vi "stage write_v2.vi"(3 "axis":u32, 4 "Incoming Handle":i32, 5 "position":dbl) -> (1 "out handle":i32)   [LabVIEW 2014]
uses:
  MCL-dll-Labview 32-bit/Madlib.dll
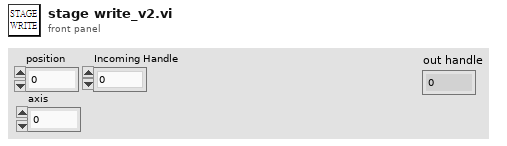
[diagram p1: front panel]
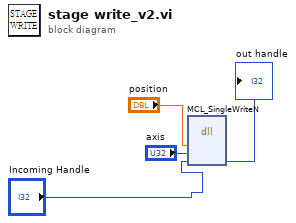
[diagram p0: block diagram]
diagram:
  n1 = dll-call lib="C:/Users/OT-hwlab/Desktop/YCC's OT/Main/Main-Stage-Based/SubVI-Stage-Based/MCL-dll-Labview 32-bit/Madlib.dll" fn="MCL_SingleWriteN"("position"="position", "axis"="axis", "handle"="Incoming Handle") -> ("handle"=→"out handle":i32)  [unwired: 6 in, 2 out]
